vi "加标模块单控对话框.vi"(11 "标题":string="加标模块") -> ()   [LabVIEW 2016, in "质控单元.lvlib"]
uses:
  <vilib>/Utility/miscctls.llb/LVPointTypeDef.ctl
panel:
  in  "流程参数读写":bool
  in  "定量":bool
  in  "排液":bool
  in  "退出":bool
  in  "柱塞泵加标":bool
  in  "搅拌":bool
  in  "进样":bool
  in  "停止":bool
  in  "加标启动":bool
  # "手动控制"
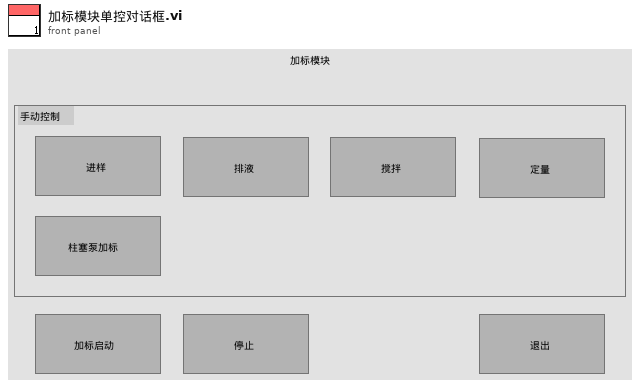
[diagram p1: front panel]
types:
  T1 = typedef "LVPointTypeDef.ctl" = cluster{"Horizontal":i16, "Vertical":i16}
  T2 = enum16{"进样", "进样停止", "排液", "排液停止", "搅拌", "搅拌停止", "定量", "定量停止"}
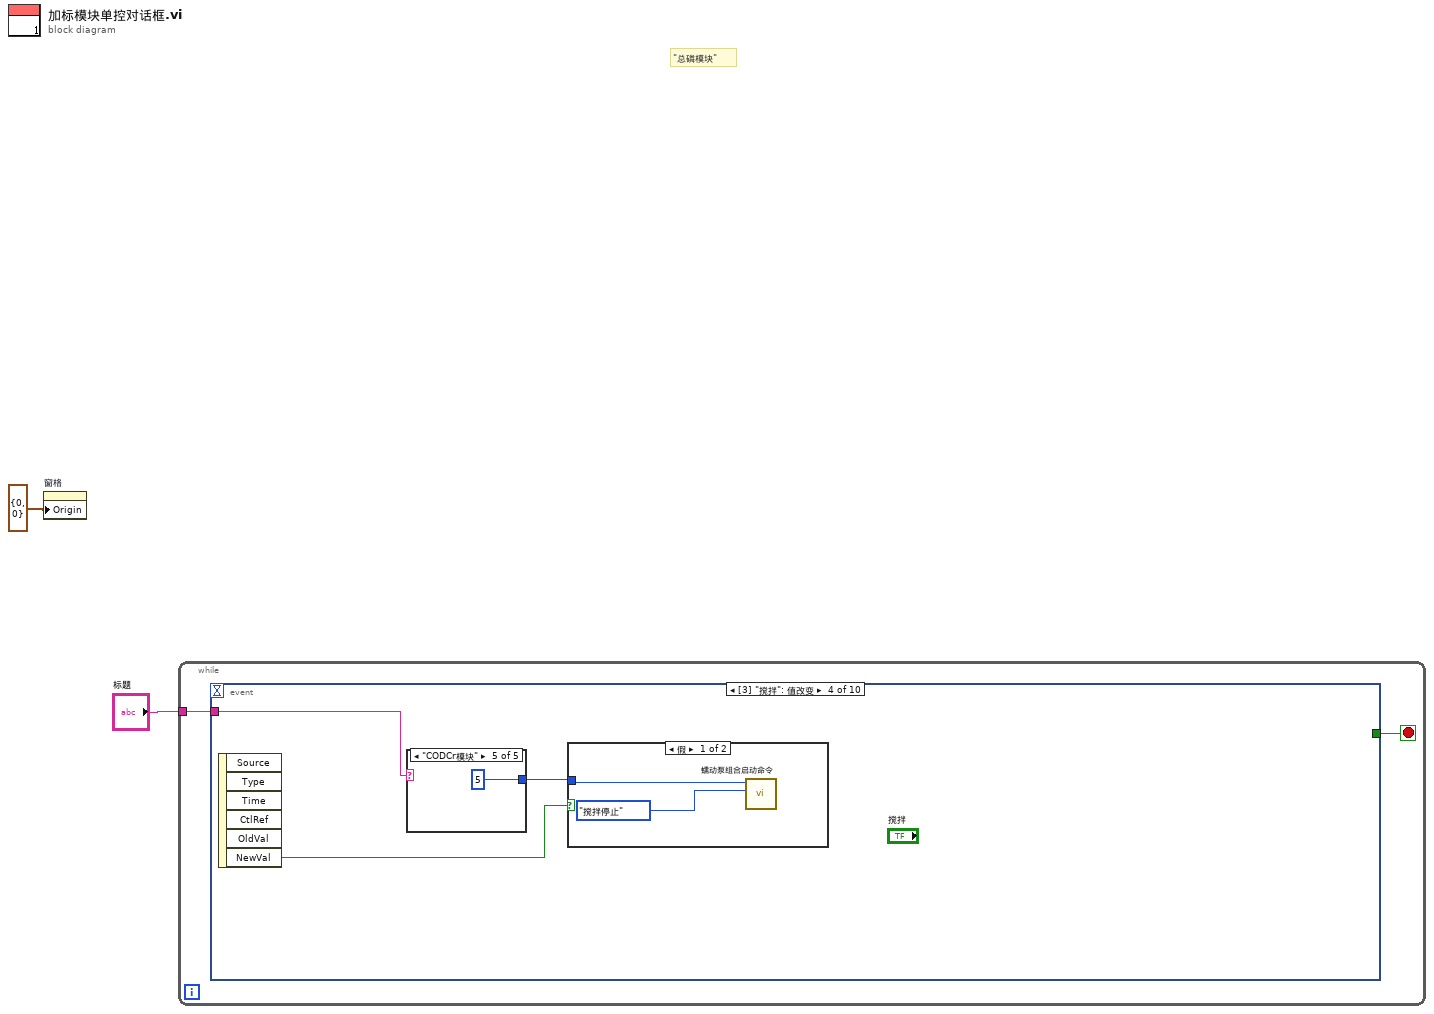
[diagram p0: block diagram]
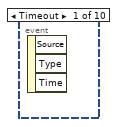
[diagram p2: hidden frame]
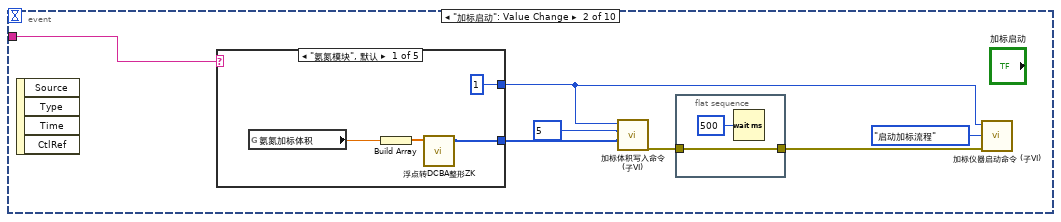
[diagram p3: hidden frame]
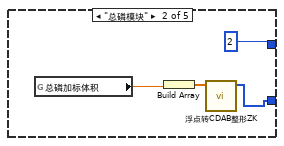
[diagram p4: hidden frame]
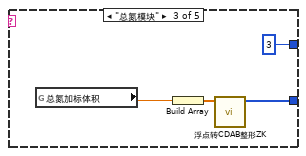
[diagram p5: hidden frame]
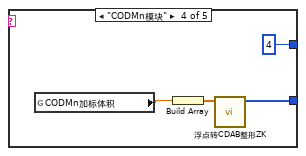
[diagram p6: hidden frame]
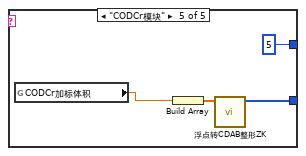
[diagram p7: hidden frame]
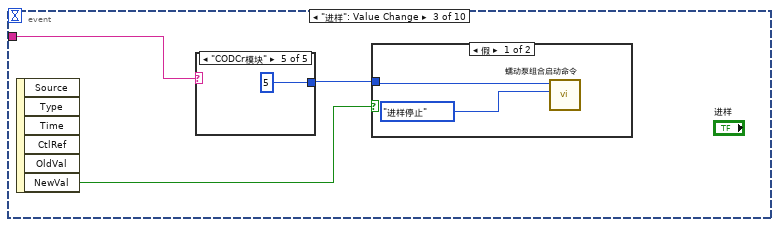
[diagram p8: hidden frame]
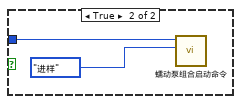
[diagram p9: hidden frame]
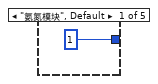
[diagram p10: hidden frame]
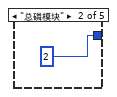
[diagram p11: hidden frame]
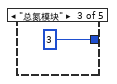
[diagram p12: hidden frame]
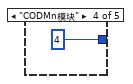
[diagram p13: hidden frame]
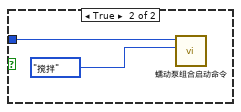
[diagram p14: hidden frame]
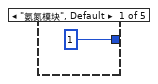
[diagram p15: hidden frame]
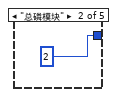
[diagram p16: hidden frame]
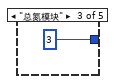
[diagram p17: hidden frame]
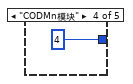
[diagram p18: hidden frame]
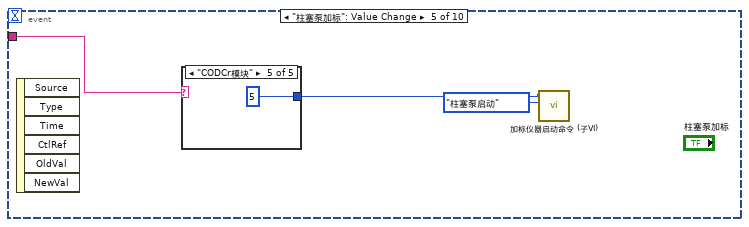
[diagram p19: hidden frame]
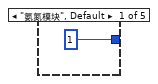
[diagram p20: hidden frame]
diagram:
  # "\"总磷模块\""
  n1 = property on="窗格" class="Pane"("Origin"=T1 {"Horizontal"=0, "Vertical"=0} ("原点")) -> ()  [unwired: 2 in, 2 out]
  n2 = while {
    tunnel: "标题" -> [w3]
    stop <- w4 stop-if-true
    n3 = event shown="[3] \"搅拌\": 值改变" {
      selector: _ -> [_ _ _ _ _ _ _ _ _ _]
      dyn-events: _ -> [_ _ _ _ _ _ _ _ _ _]
      timeout: _ -> [_ _ _ _ _ _ _ _ _ _]
      tunnel: [_ _ _ _ _ _ _ _ _ TRUE] -> w4
      tunnel: w3 -> [_ w11 w36 w48 w60 w68 w80 w100 w106 w108]
      event Timeout {
        n4 = event-data() -> ()  [unwired: 1 in, 3 out]
      }
      event "加标启动": Value Change {
        n5 = event-data() -> ()  [unwired: 1 in, 4 out]
        n6 = case shown="\"氨氮模块\", 默认" w11 {
          tunnel: [w14 w21 w24 w28 w32] -> w5
          tunnel: [u8 1 ("Slave ID") u8 2 ("Slave ID") u8 3 ("Slave ID") u8 4 ("Slave ID") u8 5 ("Slave ID")] -> w7
          frame "氨氮模块", Default {
            n7 = global read "加标回收状态全局变量.vi" "氨氮加标体积"() -> (w16:dbl)
            n8 = Build Array(w16) -> (w15:dbl[])
            n9 = call "浮点转DCBA整形ZK.vi"("浮点数"=w15) -> ("DCBA整形输出"=w14:u16[])  [unwired: 10 in]
          }
          frame "总磷模块" {
            n10 = global read "加标回收状态全局变量.vi" "总磷加标体积"() -> (w19:dbl)
            n11 = Build Array(w19) -> (w18:dbl[])
            n12 = call "浮点转CDAB整形ZK.vi"("浮点数"=w18) -> ("CDAB整形输出"=w21:u16[])  [unwired: 10 in]
          }
          frame "总氮模块" {
            n13 = global read "加标回收状态全局变量.vi" "总氮加标体积"() -> (w22:dbl)
            n14 = Build Array(w22) -> (w25:dbl[])
            n15 = call "浮点转CDAB整形ZK.vi"("浮点数"=w25) -> ("CDAB整形输出"=w24:u16[])  [unwired: 10 in]
          }
          frame "CODMn模块" {
            n16 = global read "加标回收状态全局变量.vi" "CODMn加标体积"() -> (w26:dbl)
            n17 = Build Array(w26) -> (w29:dbl[])
            n18 = call "浮点转CDAB整形ZK.vi"("浮点数"=w29) -> ("CDAB整形输出"=w28:u16[])  [unwired: 10 in]
          }
          frame "CODCr模块" {
            n19 = global read "加标回收状态全局变量.vi" "CODCr加标体积"() -> (w30:dbl)
            n20 = Build Array(w30) -> (w33:dbl[])
            n21 = call "浮点转CDAB整形ZK.vi"("浮点数"=w33) -> ("CDAB整形输出"=w32:u16[])  [unwired: 10 in]
          }
        }
        n22 = call "加标体积写入命令 (子VI).vi"("values"=w5, "starting address"=u16 5, "Slave ID"=w7) -> ("错误输出"=w8:errorcluster)  [unwired: 8 in]
        n23 = flat-sequence {
          tunnel: w8 -> [w12]
          tunnel: [w12] -> w9
          frame #0 {
            n24 = Wait (ms)(milliseconds to wait=u32 500 ("等待时间（毫秒）")) -> ()  [unwired: 1 out]
          }
        }
        n25 = call "加标仪器启动命令 (子VI).vi"("错误输入（无错误）"=w9, "启动命令"=enum16{"启动水样流程", "启动加标流程", "排液", "停止"}."启动加标流程", "仪器"=w7) -> ()  [unwired: 8 in, 1 out]
      }
      event "进样": Value Change {
        n26 = event-data() -> ("NewVal"=w34:bool)  [unwired: 1 in, 5 out]
        n27 = case shown="\"CODCr模块\"" w36 {
          tunnel: [u8 1 ("Slave ID") u8 2 ("Slave ID") u8 3 ("Slave ID") u8 4 ("Slave ID") u8 5 ("Slave ID")] -> w35
          frame "氨氮模块", Default {
          }
          frame "总磷模块" {
          }
          frame "总氮模块" {
          }
          frame "CODMn模块" {
          }
          frame "CODCr模块" {
          }
        }
        n28 = case shown="假" w34 {
          tunnel: w35 -> [w37 w40]
          frame False {
            n29 = call "蠕动泵组合启动命令.vi"("控制方式"=T2."进样停止", "仪器"=w37) -> ()  [unwired: 9 in, 1 out]
          }
          frame True {
            n30 = call "蠕动泵组合启动命令.vi"("控制方式"=T2."进样", "仪器"=w40) -> ()  [unwired: 9 in, 1 out]
          }
        }
      }
      event "搅拌": Value Change {
        n31 = event-data() -> ("NewVal"=w46:bool)  [unwired: 1 in, 5 out]
        n32 = case shown="\"CODCr模块\"" w48 {
          tunnel: [u8 1 ("Slave ID") u8 2 ("Slave ID") u8 3 ("Slave ID") u8 4 ("Slave ID") u8 5 ("Slave ID")] -> w47
          frame "氨氮模块", Default {
          }
          frame "总磷模块" {
          }
          frame "总氮模块" {
          }
          frame "CODMn模块" {
          }
          frame "CODCr模块" {
          }
        }
        n33 = case shown="假" w46 {
          tunnel: w47 -> [w49 w52]
          frame False {
            n34 = call "蠕动泵组合启动命令.vi"("控制方式"=T2."搅拌停止", "仪器"=w49) -> ()  [unwired: 9 in, 1 out]
          }
          frame True {
            n35 = call "蠕动泵组合启动命令.vi"("控制方式"=T2."搅拌", "仪器"=w52) -> ()  [unwired: 9 in, 1 out]
          }
        }
      }
      event "柱塞泵加标": Value Change {
        n36 = event-data() -> ()  [unwired: 1 in, 6 out]
        n37 = case shown="\"CODCr模块\"" w60 {
          tunnel: [u8 1 ("Slave ID") u8 2 ("Slave ID") u8 3 ("Slave ID") u8 4 ("Slave ID") u8 5 ("Slave ID")] -> w59
          frame "氨氮模块", Default {
          }
          frame "总磷模块" {
          }
          frame "总氮模块" {
          }
          frame "CODMn模块" {
          }
          frame "CODCr模块" {
          }
        }
        n38 = call "加标仪器启动命令 (子VI).vi"("启动命令"=enum16{"启动水样流程", "启动加标流程", "排液", "停止", "柱塞泵启动"}."柱塞泵启动", "仪器"=w59) -> ()  [unwired: 9 in, 1 out]
      }
      event "定量": Value Change {
        n39 = event-data() -> ("NewVal"=w66:bool)  [unwired: 1 in, 5 out]
        n40 = case shown="\"CODCr模块\"" w68 {
          tunnel: [u8 1 ("Slave ID") u8 2 ("Slave ID") u8 3 ("Slave ID") u8 4 ("Slave ID") u8 5 ("Slave ID")] -> w67
          frame "氨氮模块", Default {
          }
          frame "总磷模块" {
          }
          frame "总氮模块" {
          }
          frame "CODMn模块" {
          }
          frame "CODCr模块" {
          }
        }
        n41 = case shown="真" w66 {
          tunnel: w67 -> [w69 w72]
          frame False {
            n42 = call "蠕动泵组合启动命令.vi"("控制方式"=T2."定量停止", "仪器"=w69) -> ()  [unwired: 9 in, 1 out]
          }
          frame True {
            n43 = call "蠕动泵组合启动命令.vi"("控制方式"=T2."定量", "仪器"=w72) -> ()  [unwired: 9 in, 1 out]
          }
        }
      }
      event "排液": Value Change {
        n44 = event-data() -> ("NewVal"=w78:bool)  [unwired: 1 in, 5 out]
        n45 = case shown="\"CODCr模块\"" w80 {
          tunnel: [u8 1 ("Slave ID") u8 2 ("Slave ID") u8 3 ("Slave ID") u8 4 ("Slave ID") u8 5 ("Slave ID")] -> w79
          frame "氨氮模块", Default {
          }
          frame "总磷模块" {
          }
          frame "总氮模块" {
          }
          frame "CODMn模块" {
          }
          frame "CODCr模块" {
          }
        }
        n46 = case shown="真" w78 {
          tunnel: w79 -> [w81 w84]
          frame False {
            n47 = call "蠕动泵组合启动命令.vi"("控制方式"=T2."排液停止", "仪器"=w81) -> ()  [unwired: 9 in, 1 out]
          }
          frame True {
            n48 = call "蠕动泵组合启动命令.vi"("控制方式"=T2."排液", "仪器"=w84) -> ()  [unwired: 9 in, 1 out]
          }
        }
      }
      event "停止": Value Change {
        n49 = event-data() -> ()  [unwired: 1 in, 5 out]
        n50 = case shown="\"CODMn模块\"" w100 {
          tunnel: [u8 1 ("Slave ID") u8 2 ("Slave ID") u8 3 ("Slave ID") u8 4 ("Slave ID") u8 5 ("Slave ID")] -> w94
          frame "氨氮模块", Default {
          }
          frame "总磷模块" {
          }
          frame "总氮模块" {
          }
          frame "CODMn模块" {
          }
          frame "CODCr模块" {
          }
        }
        n51 = call "加标仪器启动命令 (子VI).vi"("启动命令"=enum16{"启动水样流程", "启动加标流程", "排液", "停止"}."停止", "仪器"=w94) -> ("错误输出"=w93:errorcluster)  [unwired: 9 in]
        n52 = call "蠕动泵组合启动命令.vi"("Error in"=w93, "控制方式"=T2."进样停止", "仪器"=w94) -> ("error out"=w92:errorcluster)  [unwired: 8 in]
        n53 = call "蠕动泵组合启动命令.vi"("Error in"=w92, "控制方式"=T2."排液停止", "仪器"=w94) -> ("error out"=w91:errorcluster)  [unwired: 8 in]
        n54 = call "蠕动泵组合启动命令.vi"("Error in"=w91, "控制方式"=T2."搅拌停止", "仪器"=w94) -> ("error out"=w90:errorcluster)  [unwired: 8 in]
        n55 = call "蠕动泵组合启动命令.vi"("Error in"=w90, "控制方式"=T2."定量停止", "仪器"=w94) -> ()  [unwired: 8 in, 1 out]
      }
      event "流程参数读写": Value Change {
        n56 = event-data() -> ()  [unwired: 1 in, 6 out]
        n57 = call "固定站质控流程参数读取对话框.vi"("标题"=w106) -> ()  [unwired: 11 in]
      }
      event "退出": Value Change; Panel Close {
        n58 = event-data() -> ()  [unwired: 1 in, 3 out]
        n59 = Two Button Dialog(message="请确认是否退出，退出仪器将停止运行" ("消息"), 1:"N" ("F按钮名称（“取消”）"), 2:"Y" ("T按钮名称（“确定”）")) -> (T button?=w107:bool)
        n60 = case shown="真" w107 {
          tunnel: w108 -> [_ w123]
          frame False {
          }
          frame True {
            n61 = case shown="\"总氮模块\"" w123 {
              tunnel: [u8 1 ("Slave ID") u8 2 ("Slave ID") u8 3 ("Slave ID") u8 4 ("Slave ID") u8 5 ("Slave ID")] -> w113
              frame "氨氮模块", Default {
              }
              frame "总磷模块" {
              }
              frame "总氮模块" {
              }
              frame "CODMn模块" {
              }
              frame "CODCr模块" {
              }
            }
            n62 = call "加标仪器启动命令 (子VI).vi"("启动命令"=enum16{"启动水样流程", "启动加标流程", "排液", "停止"}."停止", "仪器"=w113) -> ("错误输出"=w117:errorcluster)  [unwired: 9 in]
            n63 = call "蠕动泵组合启动命令.vi"("Error in"=w117, "控制方式"=T2."进样停止", "仪器"=w113) -> ("error out"=w116:errorcluster)  [unwired: 8 in]
            n64 = call "蠕动泵组合启动命令.vi"("Error in"=w116, "控制方式"=T2."排液停止", "仪器"=w113) -> ("error out"=w115:errorcluster)  [unwired: 8 in]
            n65 = call "蠕动泵组合启动命令.vi"("Error in"=w115, "控制方式"=T2."搅拌停止", "仪器"=w113) -> ("error out"=w114:errorcluster)  [unwired: 8 in]
            n66 = call "蠕动泵组合启动命令.vi"("Error in"=w114, "控制方式"=T2."定量停止", "仪器"=w113) -> ()  [unwired: 8 in, 1 out]
          }
        }
      }
    }
  }
